vi "PhaseShifter demo GUI.vi"(6 "VNA ports":bool[](array[boolean])=[TRUE, FALSE, FALSE, FALSE], 8 "Error In":errorcluster, 9 "De-embedding files":path[](array[path]), 10 "Toggle 6.lvclass":refnum<class "Toggle 6.lvclass">, 11 "Vector Network Analyzer.lvclass":refnum<class "Vector Network Analyzer.lvclass">) -> (0 "Error Out":errorcluster, 2 "Toggle 6.lvclass 2":refnum<class "Toggle 6.lvclass">, 3 "Vector Network Analyzer.lvclass 2":refnum<class "Vector Network Analyzer.lvclass">)   [LabVIEW 2020]
uses:
  Instruments/Vector Network Analyzer/Vector Network Analyzer.lvclass
  Devices/Toggle 6/Toggle 6.lvclass
  PhaseShifter demo settings.ctl
  Devices/Controls/Register to Write.ctl
  <vilib>/addons/HF Network Analysis/Support VIs/Read SnP File (SnP).vi
  <vilib>/addons/HF Network Analysis/NI_HFNetworkAnalysis.lvlib
  Devices/PIC-device/PIC-Device.lvclass
panel:
  out "Error":cluster{i32[], dbl[]}[](graph) caption="Phase error vs Setting"
  out "Measured States":i32[](array[numeric])
  out "IL (dB)":cluster{i32[], "Phase target (degree)":dbl[]}[](graph) caption="Isertion Loss (dB)"
  out "Read s2p files error out":errorcluster[](array[cluster])
  out "FoM (degree/dB)":dbl format="%#.1f"
  out "Phase change (degree)":cluster{i32[], "Phase target (degree)":dbl[]}[](graph)
  in  "Settings UI":bool
  in  "Pause Button":bool
  in  "Exit Button":bool
  in  "Mode":enum32{"Automatic mode", "Manual mode"}(radio)
  in  "Phase":i32(slide)=1 caption="Phase shift setting" min=1 max=197 step=1 scale=1.0..197.0
  out "Status bar":string
  out "Time":string
  out "Phase plot":dbl[](graph)
  out "IL data":dbl[](graph)
  out "Measured avg IL":dbl
  out "Measured range of phase":dbl
  in  "Settings":T1={"States"=32, "Timeout (ms)"=250, "Frequency (MHz)"=3500.0, "IL spec (dB)"=-2.0, "Lookup table"=path "", "Demo Mode"=enum."Live mode", "Board Loss"=0.0}
  # "Digital Phase Shifter, 3.5GHz"
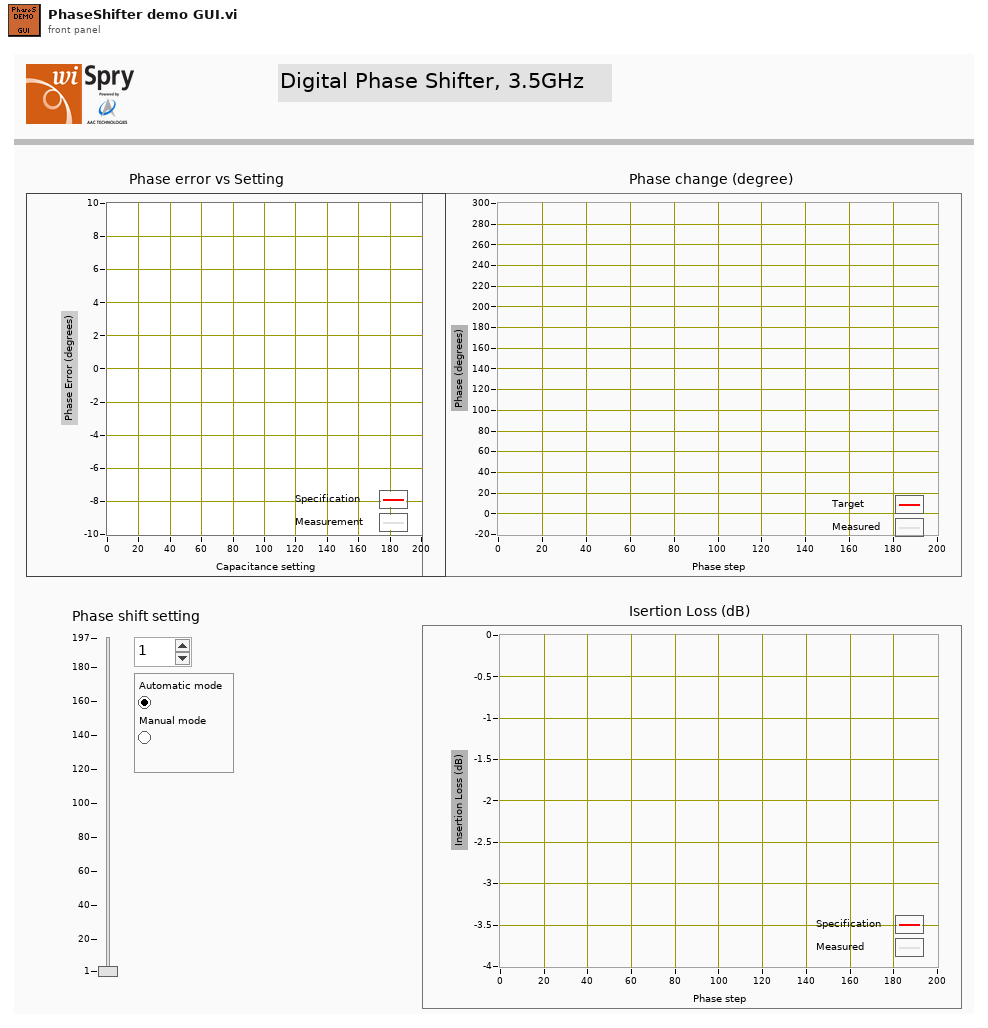
[diagram p1: front panel]
types:
  T1 = typedef "PhaseShifter demo settings.ctl" = cluster{"States":i32, "Timeout (ms)":i32, "Frequency (MHz)":dbl, "IL spec (dB)":dbl, "Lookup table":path, "Demo Mode":enum32{"Live mode", "Virtual mode"}, "Board Loss":dbl}
  T2 = enum8{"Enabled", "Disabled", "Disabled and Grayed Out"}
  T3 = typedef "PIC-Device.lvclass/Register to Write.ctl" = cluster{"Register":u32, "Value":u32, "Dev Address":u32, "Physical Adress":u32}
  T4 = typedef "Vector Network Analyzer.lvclass/Sparameter cluster.ctl" = cluster{"Frequency":dbl, "S Parameters":cdb[]}
  T5 = cluster{"Phase target (degree)":dbl[], "Phase Measured (degree)":dbl[], "Delta Phase Measured  (degree)":dbl[], "IL Measured (dB)":dbl[]}
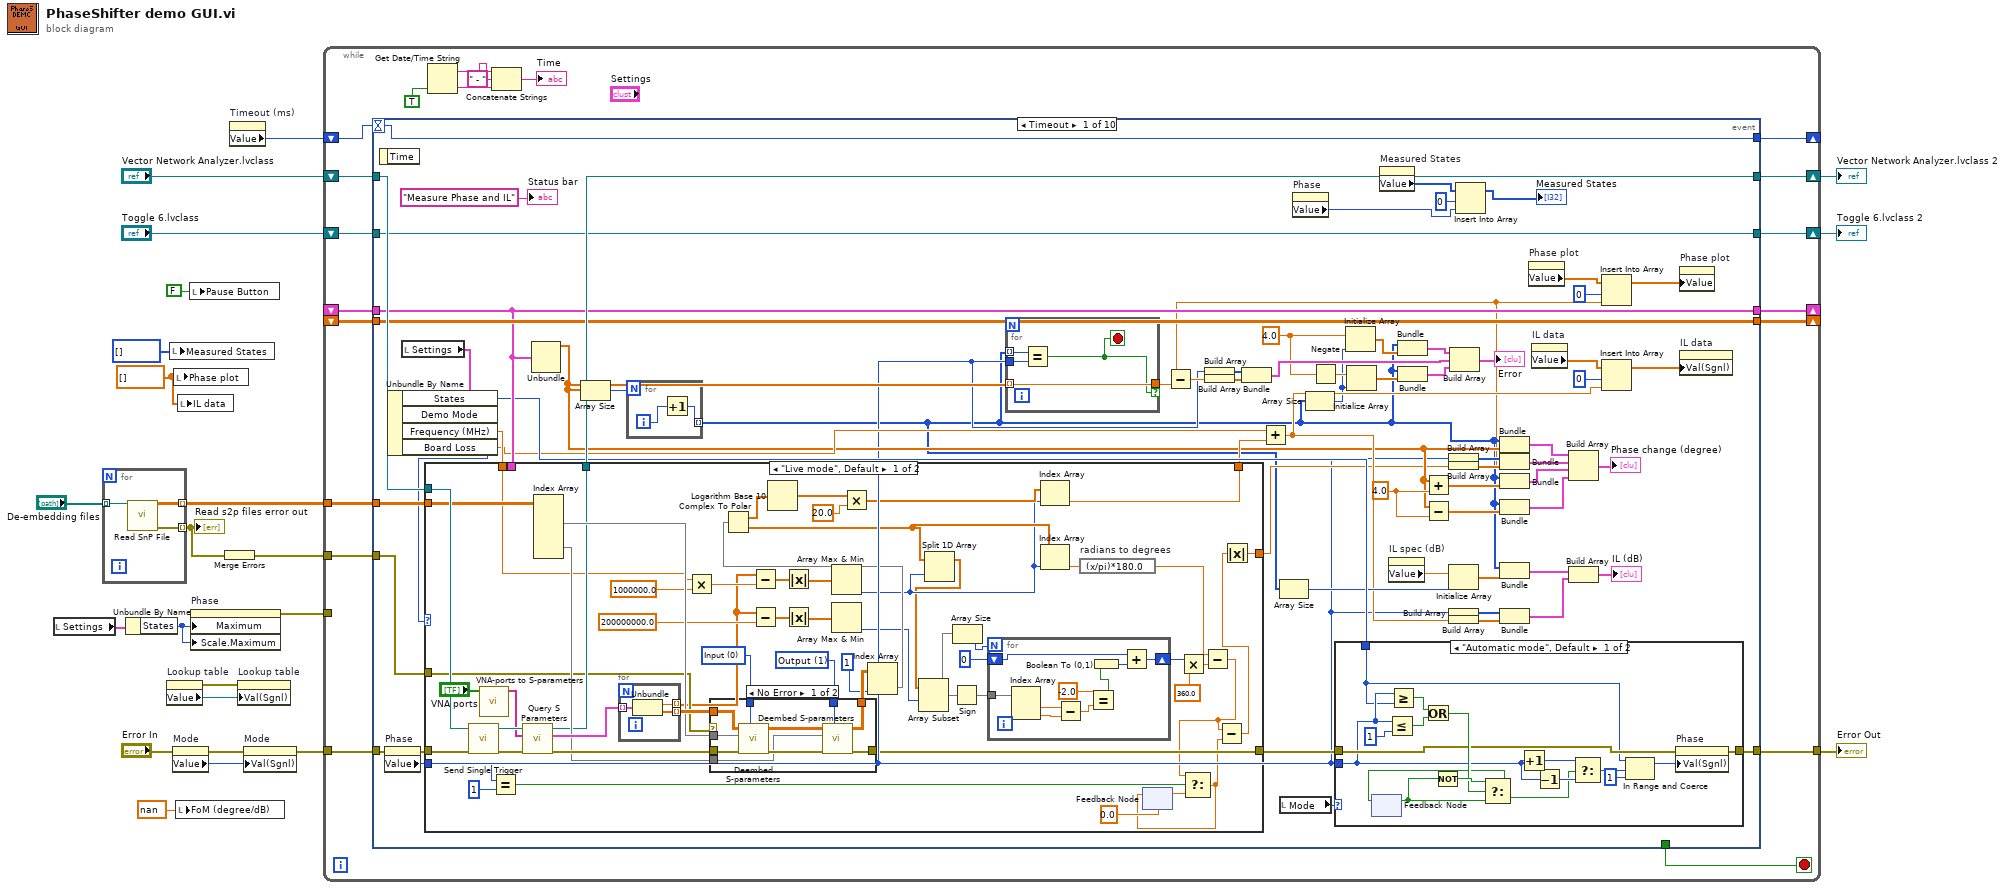
[diagram p0: block diagram]
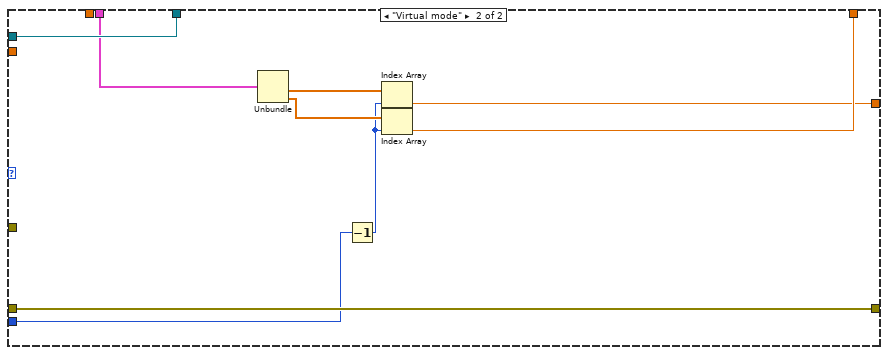
[diagram p3: hidden frame]
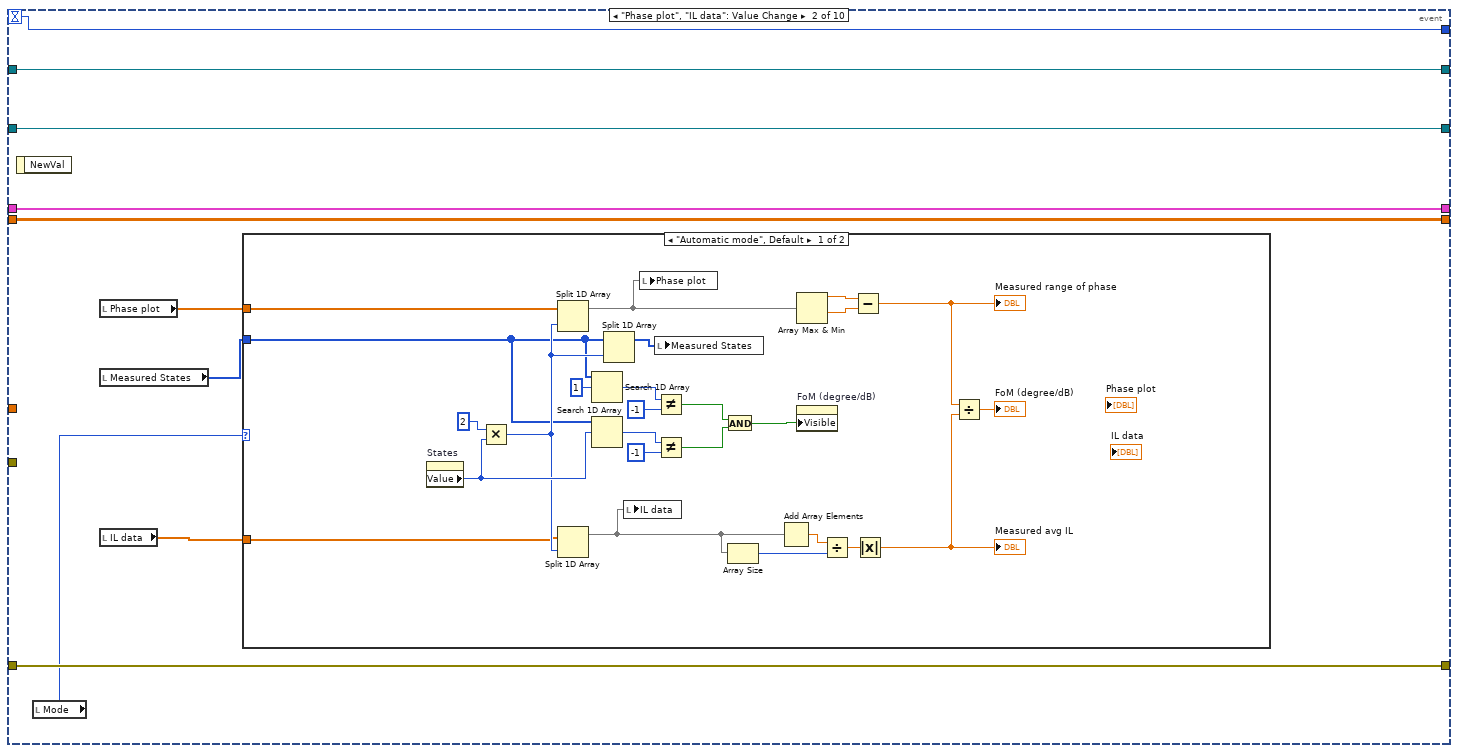
[diagram p5: hidden frame]
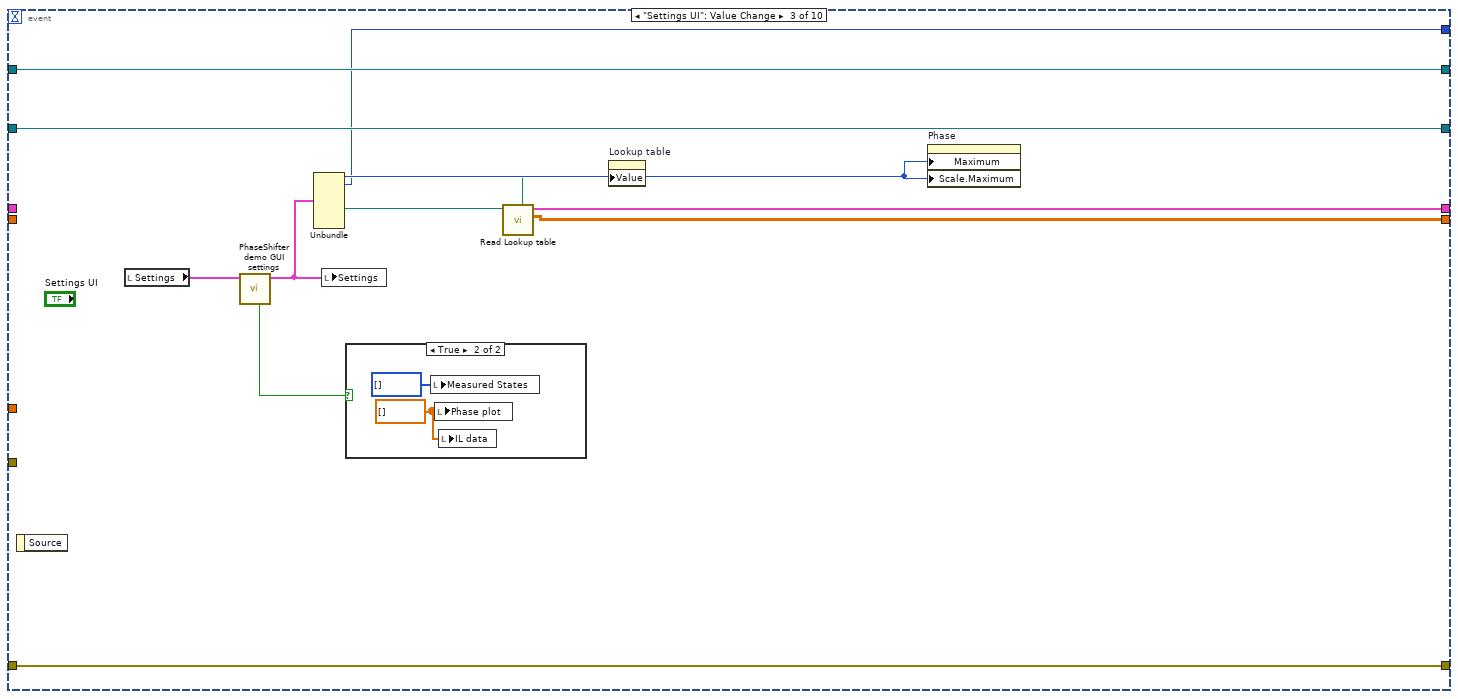
[diagram p7: hidden frame]
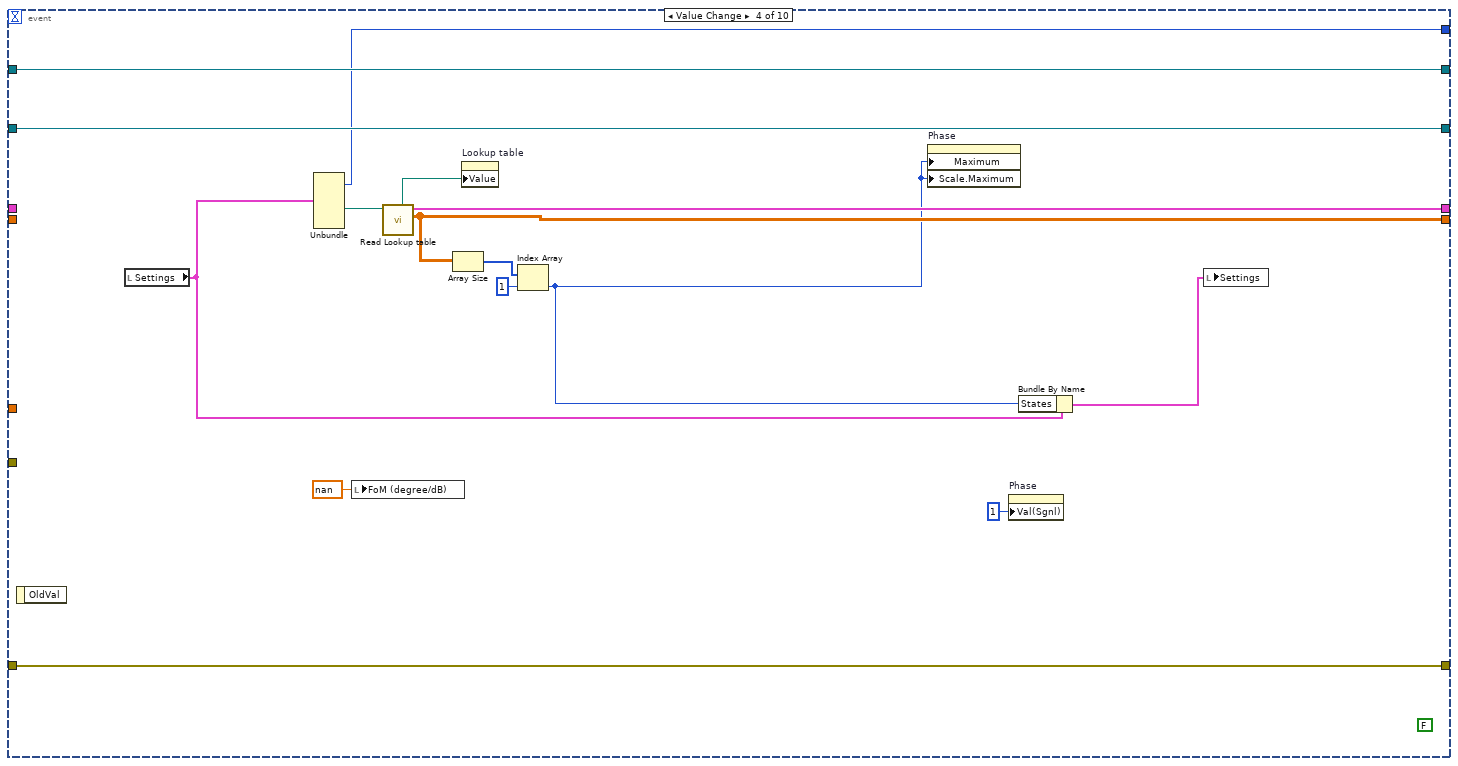
[diagram p9: hidden frame]
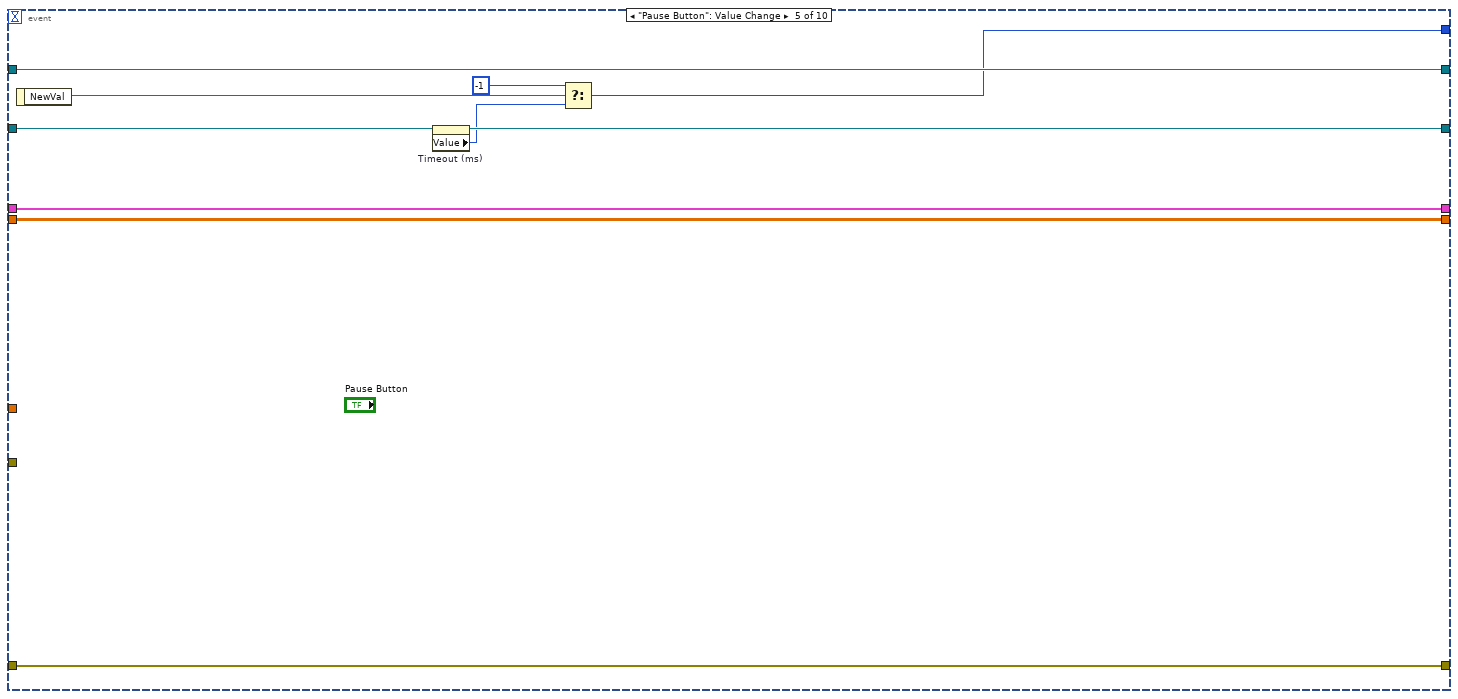
[diagram p10: hidden frame]
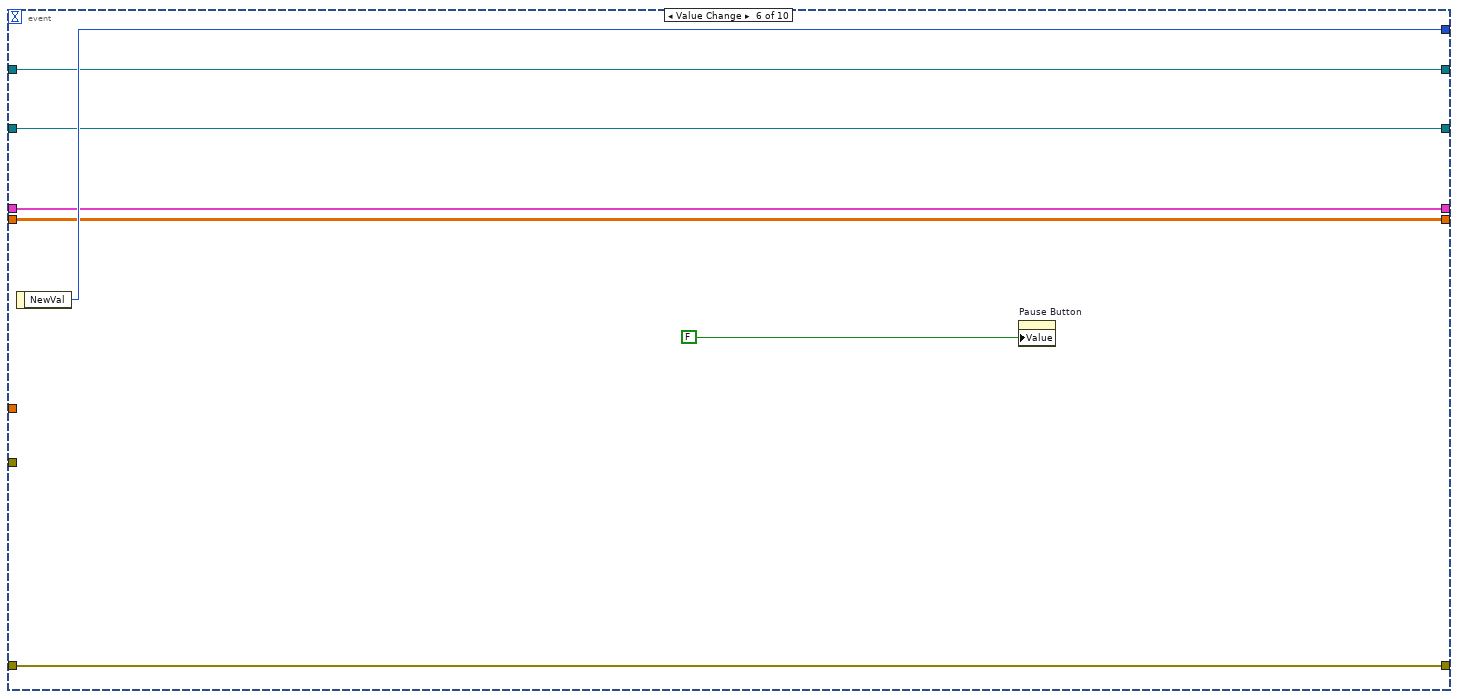
[diagram p11: hidden frame]
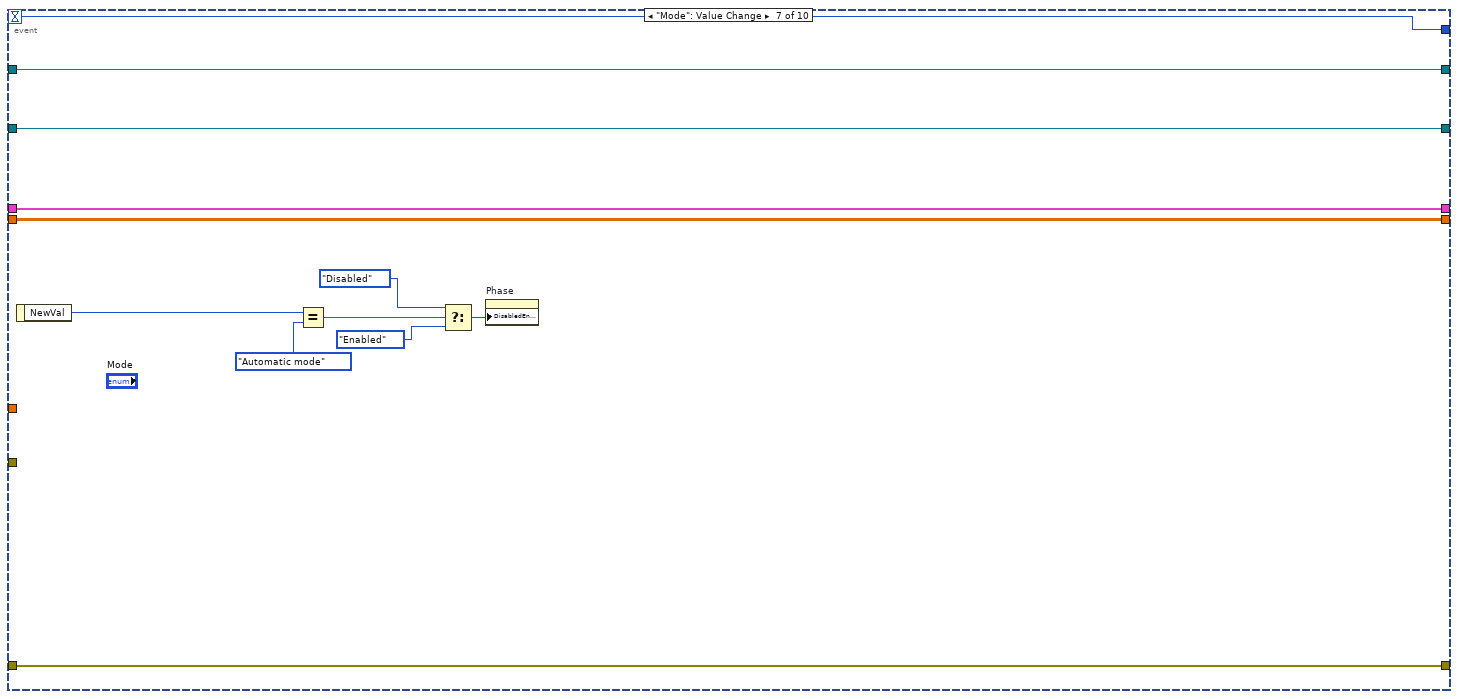
[diagram p12: hidden frame]
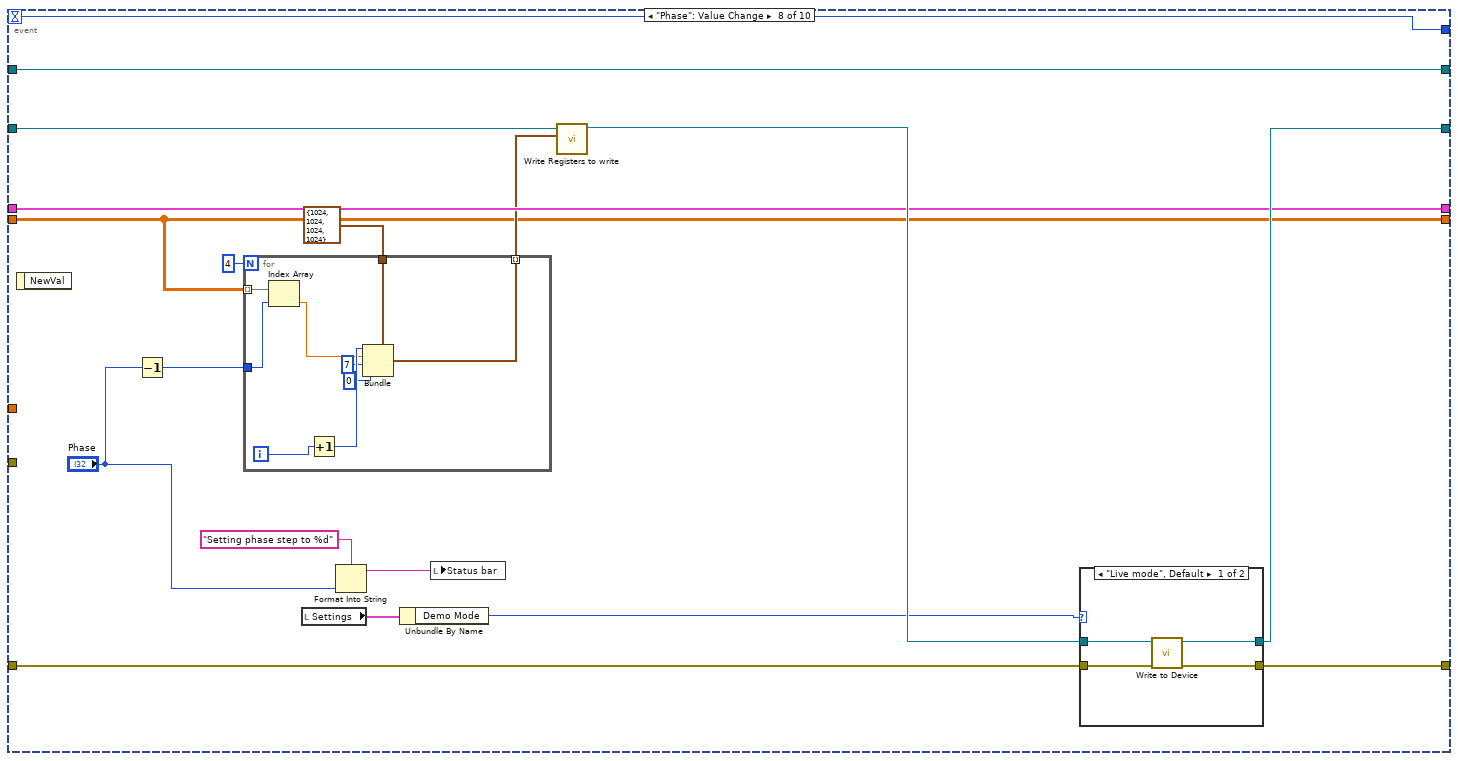
[diagram p13: hidden frame]
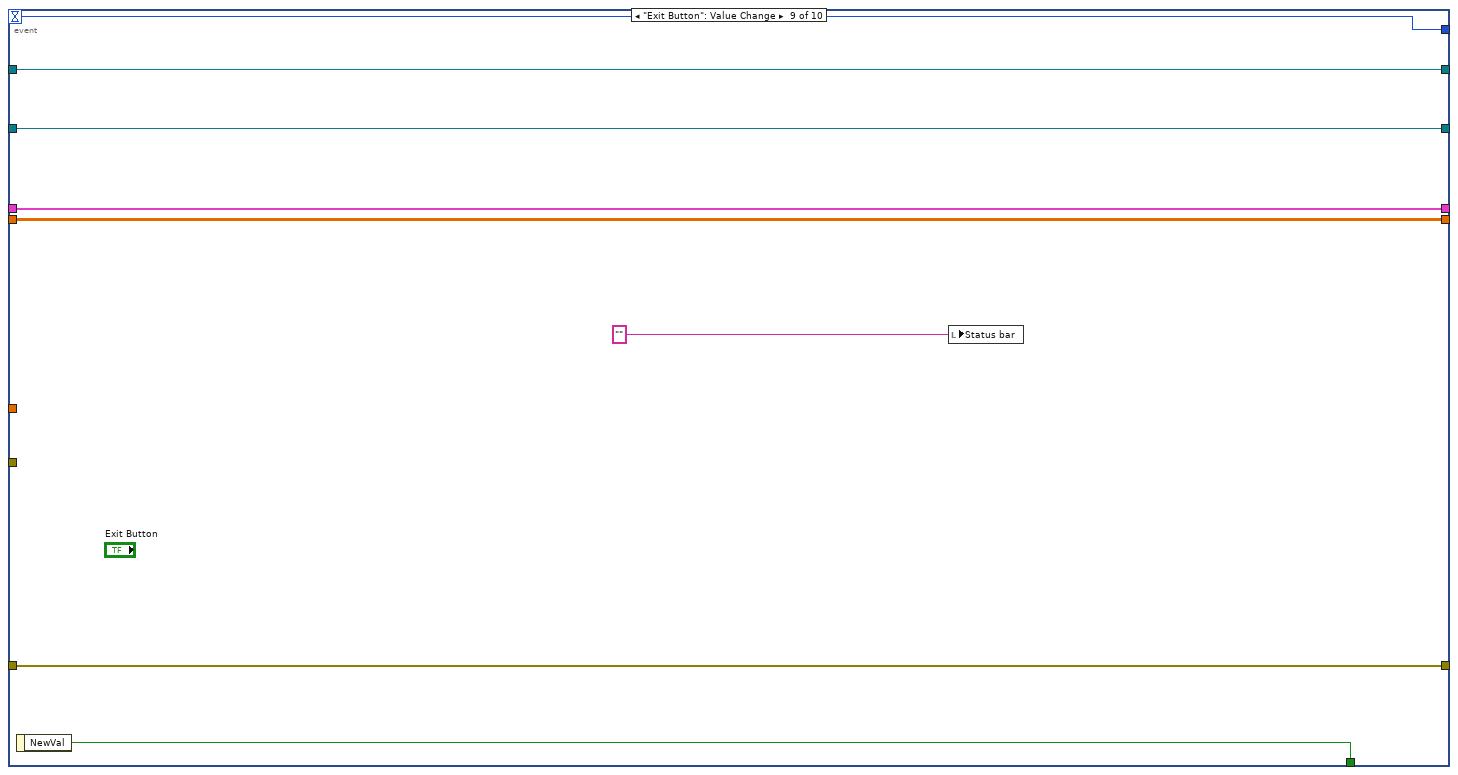
[diagram p15: hidden frame]
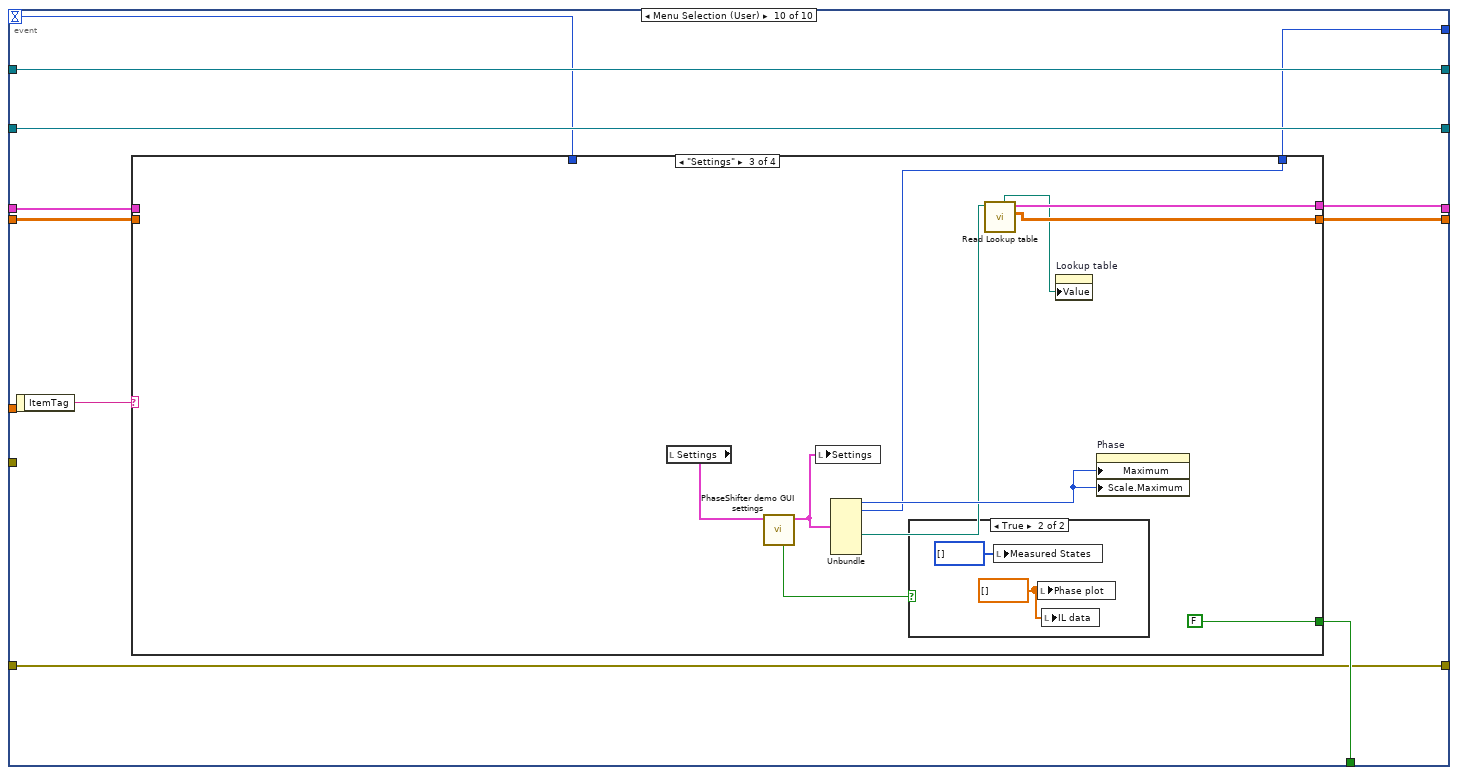
[diagram p16: hidden frame]
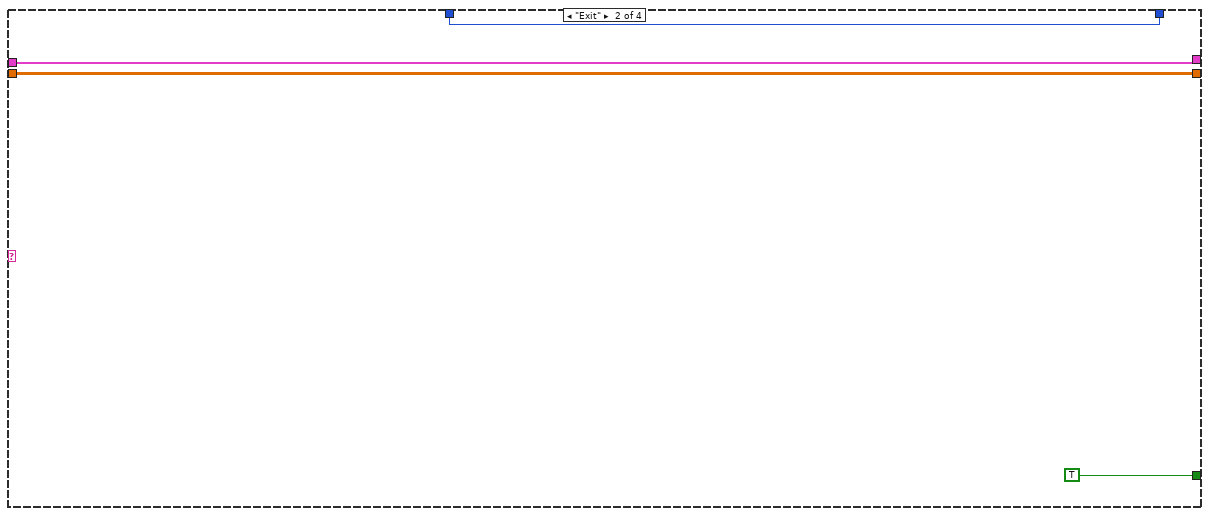
[diagram p18: hidden frame]
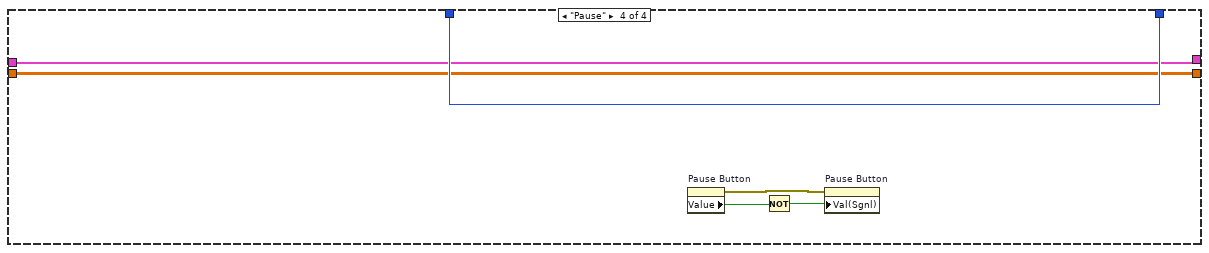
[diagram p20: hidden frame]
diagram:
  w1 = dbl[] [] ("Phase plot")
  n1 = local read "Settings"() -> (w7:T1)
  n2 = for {
    tunnel: "De-embedding files" -> [w26] mode=indexing
    tunnel: [w25] -> w10 mode=indexing
    tunnel: [w24] -> w5 mode=indexing
    n3 = call-poly <vilib>:"Read SnP File.vi"("SnP File Path"=w26) -> ("S-parameters"=w25:cdb[][], "Error Out"=w24:errorcluster)  [unwired: 11 in, 2 out]
  }
  "Read s2p files error out" <- w5
  n4 = Unbundle By Name(w7) -> ("States"=w6:i32)
  n5 = property on="Lookup table" class="Path"() -> (error out=w8:errorcluster, "Value"=w9:path)  [unwired: 2 in, 1 out]
  n6 = local write "Measured States"(i32[] [] ("Measured States")) -> ()
  n7 = property on="Mode" class="RadioBtnsControl (strict)"(error in="Error In") -> (error out=w22:errorcluster, "Value"=w23:enum32{"Automatic mode", "Manual mode"})  [unwired: 1 in, 1 out]
  n8 = local write "Phase plot"(w1) -> ()
  n9 = local write "FoM (degree/dB)"(nan ("FoM (degree/dB)")) -> ()
  n10 = local write "IL data"(w1) -> ()
  n11 = local write "Pause Button"(FALSE ("Pause Button")) -> ()
  n12 = property on="Phase" class="Slide (strict)"("Maximum"=w6, "Scale.Maximum"=w6) -> (error out=w12:errorcluster)  [unwired: 2 in, 1 out]
  n13 = Merge Errors(w5) -> (w4:errorcluster)
  n14 = property on="Timeout (ms)" class="DigNum (strict)"() -> ("Value"=w13:i32)  [unwired: 2 in, 2 out]
  n15 = property on="Lookup table" class="Path"(error in=w8, "Val(Sgnl)"=w9) -> ()  [unwired: 1 in, 2 out]
  n16 = property on="Mode" class="RadioBtnsControl (strict)"(error in=w22, "Val(Sgnl)"=w23) -> (error out=w20:errorcluster)  [unwired: 1 in, 1 out]
  n17 = while {
    tunnel: w20 -> [w45]
    shift-right: [w41] -> w18
    shift-left: "Vector Network Analyzer.lvclass" -> [w44]
    tunnel: [w43] -> w17
    shift-right: [w40] -> w15
    shift-left: "Toggle 6.lvclass" -> [w42]
    shift-right: [w38] -> _
    shift-left: w13 -> [w39]
    tunnel: w12 -> [_]
    shift-right: [w33] -> _
    shift-left: _ -> [w30]
    shift-right: [w32] -> _
    shift-left: _ -> [w31]
    tunnel: w10 -> [w29]
    tunnel: w4 -> [w27]
    stop <- w46 stop-if-true
    n18 = event shown="[0] Timeout" {
      selector: _ -> [_ _ _ _ _ _ _ _ _ _]
      dyn-events: _ -> [_ _ _ _ _ _ _ _ _ _]
      timeout: w39 -> [w108 w232 _ _ _ _ w309 w330 w355 w365]
      tunnel: [_ _ _ _ _ _ _ _ w359 w361] -> w46
      tunnel: w45 -> [w105 w231 w271 w289 w297 w303 w310 w334 w358 w360]
      tunnel: w44 -> [w113 w233 w269 w287 w299 w305 w312 w336 w357 w370]
      tunnel: [w111 w231 w271 w289 w297 w303 w310 w331 w358 w360] -> w43
      tunnel: w42 -> [w110 w234 w270 w288 w298 w304 w311 w333 w356 w369]
      tunnel: [w112 w233 w269 w287 w299 w305 w312 w336 w357 w370] -> w41
      tunnel: [w110 w234 w270 w288 w298 w304 w311 w332 w356 w369] -> w40
      tunnel: w29 -> [w107 _ _ _ _ _ _ _ _ _]
      tunnel: [w108 w232 w264 w285 w293 w306 w309 w330 w355 w364] -> w38
      tunnel: [w102 w236 w273 w290 w291 w300 w308 w325 w353 w367] -> w33
      tunnel: [w103 w235 w272 w284 w292 w301 w307 w321 w354 w366] -> w32
      tunnel: w31 -> [w103 w235 _ _ w292 w301 w307 w321 w354 w363]
      tunnel: w30 -> [w102 w236 _ _ w291 w300 w308 w325 w353 w362]
      tunnel: w27 -> [w80 _ _ _ _ _ _ _ _ _]
      event Timeout {
        w53 = 4.0
        w64 = 4.0
        n19 = event-data() -> ()  [unwired: 1 in, 1 out]
        n20 = property on="Phase" class="Slide (strict)"(error in=w105) -> (error out=w106:errorcluster, "Value"=w55:i32)  [unwired: 1 in, 1 out]
        n21 = local read "Settings"() -> (w94:T1)
        n22 = Unbundle By Name(w94) -> ("States"=w92:i32, "Demo Mode"=w93:enum32{"Live mode", "Virtual mode"}, "Frequency (MHz)"=w91:dbl, "Board Loss"=w89:dbl)
        n23 = case shown="\"Live mode\", Default" w93 {
          tunnel: w113 -> [w170 w209]
          tunnel: w106 -> [w169 w205]
          tunnel: [w162 w209] -> w112
          tunnel: [w157 w205] -> w104
          tunnel: w107 -> [w156 _]
          tunnel: w102 -> [_ w208]
          tunnel: w55 -> [w129 w202]
          tunnel: [w141 w204] -> w90
          tunnel: [w120 w203] -> w61
          tunnel: w91 -> [w154 _]
          tunnel: w80 -> [w153 _]
          frame "Live mode", Default {
            w166 = u16 1 items=["Input", "Output"] ("Deembedding Side")
            w167 = u16 0 items=["Input", "Output"] ("Deembedding Side")
            n24 = call-dynamic "Send Single Trigger.vi"("error in (no error)"=w169, "Vector Network Analyzer in"=w170) -> ("error out"=w175:errorcluster, "Vector Network Analyzer out"=w174:refnum<class "Vector Network Analyzer.lvclass">)  [unwired: 8 in]
            n25 = call "VNA-ports to S-parameters.vi"("VNA ports"="VNA ports") -> ("Sparameters (string)"=w173:string[])  [unwired: 6 in, 4 out]
            n26 = Equal?(x=w129, y=1) -> (x = y?=w127:bool)
            n27 = call-dynamic "Query S Parameters.vi"("error in (no error)"=w175, "Sparameters (string)"=w173, "Vector Network Analyzer in"=w174) -> ("error out"=w168:errorcluster, "S parameters"=w172:T4[], "Vector Network Analyzer out"=w162:refnum<class "Vector Network Analyzer.lvclass">)  [unwired: 6 in]
            n28 = Index Array(array=w156) -> (element #1=w164:cdb[][], element #2=w163:cdb[][])  [unwired: 6 in]
            n29 = for {
              tunnel: w172 -> [w200] mode=indexing
              tunnel: [w199] -> w165 mode=indexing
              tunnel: [w198] -> w130 mode=indexing
              n30 = Unbundle(w200) -> ("Frequency"=w198:dbl, "S Parameters"=w199:cdb[])
            }
            n31 = Multiply(x=w154, y=1000000.0) -> (x*y=w159:dbl)
            n32 = case shown="No Error" w153 {
              tunnel: w168 -> [w195 w197]
              tunnel: w167 -> [w193 _]
              tunnel: w166 -> [w192 _]
              tunnel: w165 -> [w191 w196]
              tunnel: w164 -> [w189 _]
              tunnel: w163 -> [w188 _]
              tunnel: [w187 w197] -> w157
              tunnel: [w186 w196] -> w155
              frame No Error {
                n33 = call <vilib>:"Deembed S-parameters.vi"("Deembedding Side"=w193, "error in (no error)"=w195, "Deembedding S-par array in"=w189, "Original S-par array in"=w191) -> ("error out"=w194:errorcluster, "Deembedded S-par array out"=w190:cdb[][])  [unwired: 6 in]
                n34 = call <vilib>:"Deembed S-parameters.vi"("Deembedding Side"=w192, "error in (no error)"=w194, "Deembedding S-par array in"=w188, "Original S-par array in"=w190) -> ("error out"=w187:errorcluster, "Deembedded S-par array out"=w186:cdb[][])  [unwired: 6 in]
              }
              frame Error {
              }
            }
            n35 = Subtract(x=w130, y=w159) -> (x-y=w161:dbl[])
            n36 = Subtract(x=w130, y=200000000.0) -> (x-y=w132:dbl[])
            n37 = Absolute Value(x=w161) -> (abs(x)=w160:dbl[])
            n38 = Absolute Value(x=w132) -> (abs(x)=w133:dbl[])
            n39 = Array Max & Min(array=w160) -> (min index (indices)=w136:i32)  [unwired: 3 out]
            n40 = Array Max & Min(array=w133) -> (min index (indices)=w131:i32)  [unwired: 3 out]
            n41 = Index Array(array=w155, index (col)=1 ("disabled index (row)")) -> (element=w145:cdb[])  [unwired: 1 in]
            n42 = Complex To Polar(r * e^(i*theta)=w145) -> (r=w152:dbl[], theta=w137:dbl[])
            n43 = Logarithm Base 10(1:w152) -> (0:w151:dbl[])
            n44 = Multiply(x=w151, y=20.0) -> (x*y=w142:dbl[])
            n45 = Split 1D Array(array=w137, index=w136) -> (first subarray=w135:dbl[])  [unwired: 1 out]
            n46 = Array Subset(array=w135, index=w131) -> (w139:dbl[])  [unwired: 1 in]
            n47 = Sign(1:w139) -> (0:w149:dbl[])
            n48 = Array Size(array=w139) -> (size(s)=w138:i32)
            n49 = for {
              N: w138 -> [_]
              tunnel: w149 -> [w185]
              shift-right: [w176] -> w143
              shift-left: 0 -> [w177]
              i -> [w184]
              n50 = Index Array(array=w185, index #1=w184) -> (element #1=w183:dbl, element #2=w182:dbl)  [unwired: 1 in]
              n51 = Subtract(x=w183, y=w182) -> (x-y=w181:dbl)
              n52 = Equal?(x=-2.0, y=w181) -> (x = y?=w178:bool)
              n53 = Boolean To (0,1)(Boolean=w178) -> (0, 1=w179:i16)
              n54 = Add(x=w177, y=w179) -> (x+y=w176:i32)
            }
            n55 = Index Array(array=w142, index=w136) -> (element=w141:dbl)
            n56 = Index Array(array=w137, index=w136) -> (element=w140:dbl)
            n57 = expression code="(x/pi)*180.0" "radians to degrees"(w140) -> (w122:dbl)
            n58 = feedback #1(0.0) -> (w124:dbl)
            n59 = Multiply(x=w143, y=360.0) -> (x*y=w147:dbl)
            n60 = Subtract(x=w122, y=w147) -> (x-y=w126:dbl)
            n61 = Select(t=w126, s=w127, f=w124) -> (s? t:f=w123:dbl)
            n62 = feedback-in #1(w123) -> ()
            n63 = Subtract(x=w126, y=w123) -> (x-y=w121:dbl)
            n64 = Absolute Value(x=w121) -> (abs(x)=w120:dbl)
          }
          frame "Virtual mode" {
            n65 = Unbundle(w208) -> ("Delta Phase Measured  (degree)"=w207:dbl[], "IL Measured (dB)"=w206:dbl[])  [unwired: 2 out]
            n66 = Decrement(x=w202) -> (x-1=w201:i32)
            n67 = Index Array(array=w207, index=w201) -> (element=w203:dbl)
            n68 = Index Array(array=w206, index=w201) -> (element=w204:dbl)
          }
        }
        n69 = Unbundle(w102) -> ("Phase target (degree)"=w63:dbl[])  [unwired: 3 out]
        n70 = Array Size(array=w63) -> (size(s)=w99:i32)
        n71 = for {
          N: w99 -> [_]
          tunnel: [w118] -> w48 mode=indexing
          i -> [w119]
          n72 = Increment(x=w119) -> (x+1=w118:i32)
        }
        n73 = for {
          tunnel: w48 -> [w117] mode=indexing
          tunnel: w55 -> [w116]
          tunnel: w63 -> [w115] mode=indexing
          tunnel: [w115] -> w62 if=w114
          stop <- w114 stop-if-true
          n74 = Equal?(x=w117, y=w116) -> (x = y?=w114:bool)
        }
        n75 = Subtract(x=w61, y=w62) -> (x-y=w57:dbl)
        n76 = Build Array(w55) -> (w56:i32[])
        n77 = Build Array(w57) -> (w58:dbl[])
        n78 = Bundle(w56, w58) -> (w54:cluster{i32[], dbl[]})  [unwired: 1 in]
        n79 = Add(x=w89, y=w90) -> (x+y=w76:dbl)
        n80 = Array Size(array=w48) -> (size(s)=w81:i32)
        n81 = local read "Mode"() -> (w109:enum32{"Automatic mode", "Manual mode"})
        n82 = property on="Phase" class="Slide (strict)"() -> ("Value"=w69:i32)  [unwired: 2 in, 2 out]
        n83 = Array Size(array=w48) -> (size(s)=w47:i32)
        n84 = Negate(x=w53) -> (-x=w51:dbl)
        n85 = case shown="\"Automatic mode\", Default" w109 {
          tunnel: w104 -> [w215 w226]
          tunnel: [w223 w226] -> w111
          tunnel: w55 -> [w214 _]
          tunnel: w92 -> [w210 _]
          frame "Automatic mode", Default {
            n86 = feedback #2() -> (w221:bool)  [unwired: 1 in]
            n87 = Less Or Equal?(x=w214, y=1) -> (x <= y?=w218:bool)
            n88 = Greater Or Equal?(x=w214, y=w210) -> (x >= y?=w219:bool)
            n89 = Or(x=w219, y=w218) -> (x .or. y?=w217:bool)
            n90 = Not(x=w221) -> (.not. x?=w222:bool)
            n91 = Select(t=w222, s=w217, f=w221) -> (s? t:f=w216:bool)
            n92 = feedback-in #2(w216) -> ()
            n93 = Increment(x=w214) -> (x+1=w224:i32)
            n94 = Decrement(x=w214) -> (x-1=w225:i32)
            n95 = Select(t=w224, s=w216, f=w225) -> (s? t:f=w213:i32)
            n96 = In Range and Coerce(upper limit=w210, x=w213, lower limit=1) -> (coerced(x)=w212:i32)  [unwired: 1 out]
            n97 = property on="Phase" class="Slide (strict)"(error in=w215, "Val(Sgnl)"=w212) -> (error out=w223:errorcluster)  [unwired: 1 in, 1 out]
          }
          frame "Manual mode" {
          }
        }
        n98 = Initialize Array(w53, w47) -> (w52:dbl[])
        n99 = Initialize Array(w51, w47) -> (w50:dbl[])
        n100 = property on="Measured States" class="Arr (strict)"() -> ("Value"=w71:i32[])  [unwired: 2 in, 2 out]
        n101 = property on="IL spec (dB)" class="DigNum (strict)"() -> ("Value"=w82:dbl)  [unwired: 2 in, 2 out]
        n102 = Bundle(w48, w52) -> (w60:cluster{i32[], dbl[]})  [unwired: 1 in]
        n103 = Bundle(w48, w50) -> (w59:cluster{i32[], dbl[]})  [unwired: 1 in]
        n104 = Add(x=w63, y=w64) -> (x+y=w66:dbl[])
        n105 = Subtract(x=w63, y=w64) -> (x-y=w65:dbl[])
        n106 = Build Array(w55) -> (w97:i32[])
        n107 = Build Array(w61) -> (w96:dbl[])
        n108 = Initialize Array(w82, w81) -> (w83:dbl[])
        n109 = Build Array(w55) -> (w87:i32[])
        n110 = Build Array(w76) -> (w88:dbl[])
        n111 = Build Array(w60, w54, w59) -> (→"Error":cluster{i32[], dbl[]}[])
        n112 = Insert Into Array(array=w71, index=0, new element=w69) -> (→"Measured States":i32[])
        n113 = Bundle(w48, "Phase target (degree)"=w63) -> (w100:cluster{i32[], "Phase target (degree)":dbl[]})  [unwired: 1 in]
        n114 = Bundle(w97, w96) -> (w101:cluster{i32[], dbl[]})  [unwired: 1 in]
        n115 = Bundle(w48, w66) -> (w68:cluster{i32[], dbl[]})  [unwired: 1 in]
        n116 = Bundle(w48, w65) -> (w67:cluster{i32[], dbl[]})  [unwired: 1 in]
        n117 = Bundle(w48, w83) -> (w86:cluster{i32[], dbl[]})  [unwired: 1 in]
        n118 = Bundle(w87, w88) -> (w85:cluster{i32[], dbl[]})  [unwired: 1 in]
        n119 = property on="Phase plot" class="WFGraph (strict)"() -> ("Value"=w79:dbl[])  [unwired: 2 in, 2 out]
        n120 = property on="IL data" class="WFGraph (strict)"() -> ("Value"=w77:dbl[])  [unwired: 2 in, 2 out]
        n121 = Build Array(w100, w101, w68, w67) -> (→"Phase change (degree)":cluster{i32[], "Phase target (degree)":dbl[]}[])
        n122 = Build Array(w86, w85) -> (→"IL (dB)":cluster{i32[], dbl[]}[])
        n123 = Insert Into Array(array=w79, index=0, new element=w61) -> (w78:dbl[])
        n124 = Insert Into Array(array=w77, index=0, new element=w76) -> (w75:dbl[])
        n125 = property on="Phase plot" class="WFGraph (strict)"("Value"=w78) -> ()  [unwired: 2 in, 2 out]
        n126 = property on="IL data" class="WFGraph (strict)"("Val(Sgnl)"=w75) -> ()  [unwired: 2 in, 2 out]
        "Status bar" <- "Measure Phase and IL" ("Status bar")
      }
      event "Phase plot", "IL data": Value Change {
        n127 = event-data() -> ()  [unwired: 1 in, 1 out]
        n128 = local read "Mode"() -> (w230:enum32{"Automatic mode", "Manual mode"})
        n129 = local read "Phase plot"() -> (w227:dbl[])
        n130 = local read "Measured States"() -> (w229:i32[])
        n131 = local read "IL data"() -> (w228:dbl[])
        n132 = case shown="\"Automatic mode\", Default" w230 {
          tunnel: w229 -> [w239 _]
          tunnel: w228 -> [w238 _]
          tunnel: w227 -> [w237 _]
          frame "Automatic mode", Default {
            n133 = property on="States" class="DigNum (strict)"() -> ("Value"=w249:i32)  [unwired: 2 in, 2 out]
            n134 = Multiply(x=2, y=w249) -> (x*y=w240:i32)
            n135 = Split 1D Array(array=w237, index=w240) -> (first subarray=w252:dbl[])  [unwired: 1 out]
            n136 = Split 1D Array(array=w238, index=w240) -> (first subarray=w251:dbl[])  [unwired: 1 out]
            n137 = Search 1D Array(1D array=w239, element=1) -> (index of element=w242:i32)  [unwired: 1 in]
            n138 = Search 1D Array(1D array=w239, element=w249) -> (index of element=w246:i32)  [unwired: 1 in]
            n139 = Split 1D Array(array=w239, index=w240) -> (first subarray=w241:i32[])  [unwired: 1 out]
            n140 = local write "IL data"(w251) -> ()
            n141 = local write "Phase plot"(w252) -> ()
            n142 = local write "Measured States"(w241) -> ()
            n143 = Not Equal?(x=w242, y=-1) -> (x != y?=w245:bool)
            n144 = Not Equal?(x=w246, y=-1) -> (x != y?=w244:bool)
            n145 = And(x=w245, y=w244) -> (x .and. y?=w243:bool)
            n146 = Array Size(array=w251) -> (size(s)=w258:i32)
            n147 = Add Array Elements(numeric array=w251) -> (sum=w259:dbl)
            n148 = Array Max & Min(array=w252) -> (max value=w261:dbl, min value=w260:dbl)  [unwired: 2 out]
            n149 = property on="FoM (degree/dB)" class="DigNum (strict)"("Visible"=w243) -> ()  [unwired: 2 in, 2 out]
            n150 = Divide(x=w259, y=w258) -> (x/y=w254:dbl)
            n151 = Subtract(x=w261, y=w260) -> (x-y=w257:dbl)
            "Measured range of phase" <- w257
            n152 = Absolute Value(x=w254) -> (abs(x)=w253:dbl)
            "Measured avg IL" <- w253
            n153 = Divide(x=w257, y=w253) -> (x/y=→"FoM (degree/dB)":dbl)
          }
          frame "Manual mode" {
          }
        }
      }
      event "Settings UI": Value Change {
        n154 = event-data() -> ()  [unwired: 1 in, 1 out]
        n155 = local read "Settings"() -> (w268:T1)
        n156 = call "PhaseShifter demo GUI settings.vi"("Settings"=w268) -> ("Settings 2"=w267:T1, "Reset FoM calculation 2"=w263:bool)  [unwired: 9 in]
        n157 = Unbundle(w267) -> ("States"=w265:i32, "Timeout (ms)"=w264:i32, "Lookup table"=w266:path)  [unwired: 4 out]
        n158 = local write "Settings"(w267) -> ()
        n159 = case shown="True" w263 {
          frame False {
          }
          frame True {
            w274 = dbl[] [] ("Phase plot")
            n160 = local write "Measured States"(i32[] [] ("Measured States")) -> ()
            n161 = local write "Phase plot"(w274) -> ()
            n162 = local write "IL data"(w274) -> ()
          }
        }
        n163 = call "Read Lookup table.vi"("file path (dialog if empty)"=w266) -> ("C1...C4"=w272:dbl[][], "Data"=w273:T5, "new file path (Not A Path if cancelled)"=w262:path)  [unwired: 8 in]
        n164 = property on="Lookup table" class="Path"("Value"=w262) -> ()  [unwired: 2 in, 2 out]
        n165 = property on="Phase" class="Slide (strict)"("Maximum"=w265, "Scale.Maximum"=w265) -> ()  [unwired: 2 in, 2 out]
      }
      event Value Change {
        (unwired) FALSE
        n166 = event-data() -> ()  [unwired: 1 in, 1 out]
        n167 = local read "Settings"() -> (w281:T1)
        n168 = Unbundle(w281) -> ("Timeout (ms)"=w285:i32, "Lookup table"=w286:path)  [unwired: 5 out]
        n169 = local write "FoM (degree/dB)"(nan ("FoM (degree/dB)")) -> ()
        n170 = call "Read Lookup table.vi"("file path (dialog if empty)"=w286) -> ("C1...C4"=w284:dbl[][], "Data"=w290:T5, "new file path (Not A Path if cancelled)"=w276:path)  [unwired: 8 in]
        n171 = Array Size(array=w284) -> (size(s)=w283:i32[])
        n172 = property on="Lookup table" class="Path"("Value"=w276) -> ()  [unwired: 2 in, 2 out]
        n173 = Index Array(array=w283, index=1) -> (element=w279:i32)
        n174 = property on="Phase" class="Slide (strict)"("Maximum"=w279, "Scale.Maximum"=w279) -> ()  [unwired: 2 in, 2 out]
        n175 = property on="Phase" class="Slide (strict)"("Val(Sgnl)"=1 ("Value (Signaling)")) -> ()  [unwired: 2 in, 2 out]
        n176 = Bundle By Name(cluster=w281, "States"=w279) -> (w280:T1)
        n177 = local write "Settings"(w280) -> ()
      }
      event "Pause Button": Value Change {
        n178 = event-data() -> ("NewVal"=w296:bool)  [unwired: 1 in]
        n179 = property on="Timeout (ms)" class="DigNum (strict)"() -> ("Value"=w295:i32)  [unwired: 2 in, 2 out]
        n180 = Select(t=-1, s=w296, f=w295) -> (s? t:f=w293:i32)
      }
      event Value Change {
        n181 = event-data() -> ("NewVal"=w306:i32)  [unwired: 1 in]
        n182 = property on="Pause Button" class="Bool (strict)"("Value"=FALSE ("Pause Button")) -> ()  [unwired: 2 in, 2 out]
      }
      event "Mode": Value Change {
        n183 = event-data() -> ("NewVal"=w318:enum32{"Automatic mode", "Manual mode"})  [unwired: 1 in]
        n184 = Equal?(x=w318, y=enum32{"Automatic mode", "Manual mode"}."Automatic mode") -> (x = y?=w316:bool)
        n185 = Select(t=T2."Disabled" ("Disabled"), s=w316, f=T2."Enabled" ("Disabled")) -> (s? t:f=w313:T2)
        n186 = property on="Phase" class="Slide (strict)"("DisabledEnum"=w313) -> ()  [unwired: 2 in, 2 out]
      }
      event "Phase": Value Change {
        n187 = event-data() -> ()  [unwired: 1 in, 1 out]
        n188 = Decrement(x="Phase") -> (x-1=w319:i32)
        n189 = for {
          N: 4 -> [_]
          tunnel: T3 {"Register"=1024, "Value"=1024, "Dev Address"=1024, "Physical Adress"=1024} ("Register cluster out") -> [w345]
          tunnel: [w342] -> w322 mode=indexing
          tunnel: w321 -> [w339] mode=indexing
          tunnel: w319 -> [w337]
          i -> [w344]
          n190 = Index Array(array=w339, index=w337) -> (element=w338:dbl)
          n191 = Increment(x=w344) -> (x+1=w343:i32)
          n192 = Bundle(cluster=w345, "Register"=w343, "Value"=w338, "Dev Address"=u32 7 ("Dev Adress"), "Physical Adress"=u32 0) -> (w342:T3)
        }
        n193 = local read "Settings"() -> (w327:T1)
        n194 = Format Into String(format string="Setting phase step to %d" ("Status bar"), "Phase") -> (resulting string=w328:string)  [unwired: 2 in, 1 out]
        n195 = Unbundle By Name(w327) -> ("Demo Mode"=w326:enum32{"Live mode", "Virtual mode"})
        n196 = local write "Status bar"(w328) -> ()
        n197 = call-dynamic "Write Registers to write.vi"("Registers to write"=w322, "Device in"=w333) -> ("Device out"=w335:refnum<class "Toggle 6.lvclass">)  [unwired: 9 in]
        n198 = case shown="\"Live mode\", Default" w326 {
          tunnel: w335 -> [w349 w350]
          tunnel: w334 -> [w348 w351]
          tunnel: [w347 w350] -> w332
          tunnel: [w346 w351] -> w331
          frame "Live mode", Default {
            n199 = call-dynamic "Write to Device.vi"("error in (no error)"=w348, "Device in"=w349) -> ("error out"=w346:errorcluster, "Device out"=w347:refnum<class "Toggle 6.lvclass">)  [unwired: 7 in, 1 out]
          }
          frame "Virtual mode" {
          }
        }
      }
      event "Exit Button": Value Change {
        n200 = event-data() -> ("NewVal"=w359:bool)  [unwired: 1 in]
        n201 = local write "Status bar"("" ("Status bar")) -> ()
      }
      event Menu Selection (User) {
        n202 = event-data() -> ("ItemTag"=w368:string)  [unwired: 1 in]
        n203 = case shown="\"Settings\"" w368 {
          tunnel: [_ TRUE FALSE _] -> w361
          tunnel: [w373 w376 w380 w392] -> w364
          tunnel: w365 -> [w373 w376 _ w392]
          tunnel: [w371 w374 w382 w390] -> w367
          tunnel: [w372 w375 w381 w391] -> w366
          tunnel: w363 -> [w372 w375 _ w391]
          tunnel: w362 -> [w371 w374 _ w390]
          frame Default {
          }
          frame "Exit" {
          }
          frame "Settings" {
            n204 = local read "Settings"() -> (w386:T1)
            n205 = call "PhaseShifter demo GUI settings.vi"("Settings"=w386) -> ("Settings 2"=w385:T1, "Reset FoM calculation 2"=w379:bool)  [unwired: 9 in]
            n206 = local write "Settings"(w385) -> ()
            n207 = Unbundle(w385) -> ("States"=w384:i32, "Timeout (ms)"=w380:i32, "Lookup table"=w383:path)  [unwired: 4 out]
            n208 = case shown="True" w379 {
              frame False {
              }
              frame True {
                w388 = dbl[] [] ("Phase plot")
                n209 = local write "Measured States"(i32[] [] ("Measured States")) -> ()
                n210 = local write "Phase plot"(w388) -> ()
                n211 = local write "IL data"(w388) -> ()
              }
            }
            n212 = call "Read Lookup table.vi"("file path (dialog if empty)"=w383) -> ("C1...C4"=w381:dbl[][], "Data"=w382:T5, "new file path (Not A Path if cancelled)"=w378:path)  [unwired: 8 in]
            n213 = property on="Lookup table" class="Path"("Value"=w378) -> ()  [unwired: 2 in, 2 out]
            n214 = property on="Phase" class="Slide (strict)"("Maximum"=w384, "Scale.Maximum"=w384) -> ()  [unwired: 2 in, 2 out]
          }
          frame "Pause" {
            n215 = property on="Pause Button" class="Bool (strict)"() -> (error out=w393:errorcluster, "Value"=w395:bool)  [unwired: 2 in, 1 out]
            n216 = Not(x=w395) -> (.not. x?=w394:bool)
            n217 = property on="Pause Button" class="Bool (strict)"(error in=w393, "Val(Sgnl)"=w394) -> ()  [unwired: 1 in, 2 out]
          }
        }
      }
    }
    n218 = Get Date/Time String(want seconds? (F)=TRUE) -> (date string=w36:string, time string=w37:string)  [unwired: 2 in]
    n219 = Concatenate Strings(w36, " - " ("string"), w37) -> (→"Time":string)
  }
  "Vector Network Analyzer.lvclass 2" <- w18
  "Error Out" <- w17
  "Toggle 6.lvclass 2" <- w15
